vi "RichToFlatni_measurementlink_pinmap_v1_ChannelMapping.vi"(5 "OutputClusterType":T1, 11 "InputCluster":T2) -> (3 "OutputCluster":T1)   [LabVIEW 2020, in "Measurement Plugin Pin Map Client.lvlib"]
uses:
  Measurement Plugin Pin Map Client.lvlib
  ni_measurementlink_pinmap_v1_ChannelMapping.ctl
  ni_measurementlink_pinmap_v1_ChannelMapping_Flat.ctl
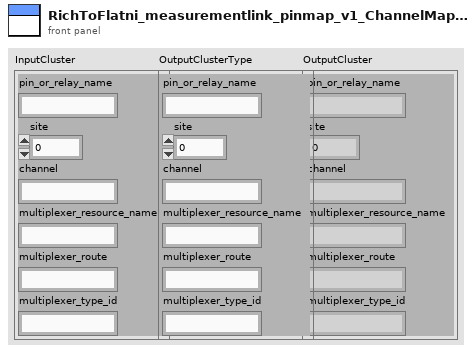
[diagram p1: front panel]
types:
  T1 = typedef "Measurement Plugin Pin Map Client.lvlib/ni_measurementlink_pinmap_v1_ChannelMapping_Flat.ctl" = cluster{"pin_or_relay_name":string, "site":i32, "channel":string, "multiplexer_resource_name":string, "multiplexer_route":string, "multiplexer_type_id":string}
  T2 = typedef "Measurement Plugin Pin Map Client.lvlib/ni_measurementlink_pinmap_v1_ChannelMapping.ctl" = cluster{"pin_or_relay_name":string, "site":i32, "channel":string, "multiplexer_resource_name":string, "multiplexer_route":string, "multiplexer_type_id":string}
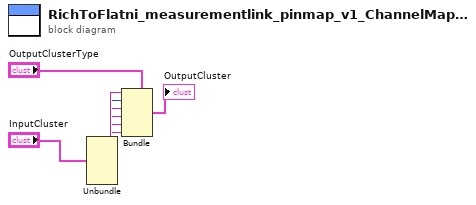
[diagram p0: block diagram]
diagram:
  n1 = Unbundle "Unbundle"("InputCluster") -> ("pin_or_relay_name"=w6:string, "site"=w5:i32, "channel"=w4:string, "multiplexer_resource_name"=w3:string, "multiplexer_route"=w2:string, "multiplexer_type_id"=w1:string)
  n2 = Bundle "Bundle"(cluster="OutputClusterType", "pin_or_relay_name"=w6, "site"=w5, "channel"=w4, "multiplexer_resource_name"=w3, "multiplexer_route"=w2, "multiplexer_type_id"=w1) -> (→"OutputCluster":T1)
